vi "correctwaveformsizetemp.vi"(0 "new sampling frequency (Hz)":dbl, 1 "start":bool, 2 "reference waveforms to":string, 3 "Analog waveforms in":waveform(dbl)[](array[waveform]), 4 "stop":bool, 5 "Digital waveforms in":digitalwaveform[](array[waveform])) -> (6 "analog wf out":waveform(dbl)[](array[waveform]), 7 "Digital wf out":digitalwaveform[](array[waveform]), 8 "measpoints":i32)   [LabVIEW 2015]
uses:
  generateRampedSquareWave.vi
  waveformformfile.vi
  <vilib>/Waveform/DWDTOps.llb/DWDT Digital Size.vi
  digitalwffromfile.vi
  <vilib>/Waveform/DWDTOps.llb/DWDT Analog to Digital.vi
  <vilib>/Waveform/DWDTOps.llb/DWDT Append Digital Samples.vi
  <vilib>/Waveform/DWDTOps.llb/DWDT Get Waveform Subset.vi
  <vilib>/Waveform/WDTOps.llb/WDT Get Waveform Subset DBL.vi
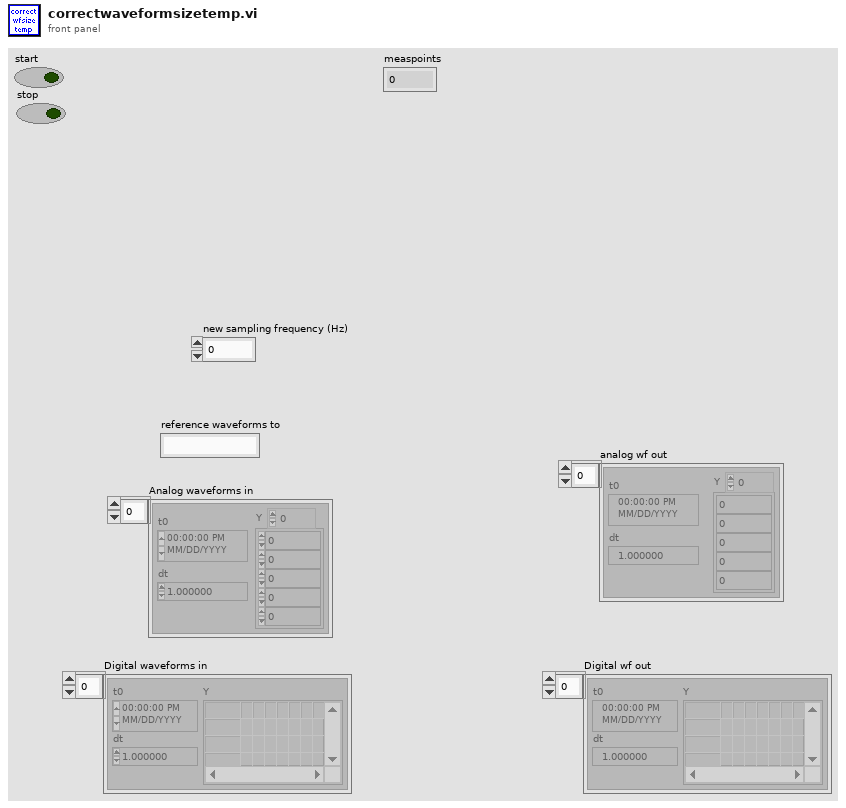
[diagram p1: front panel]
types:
  T1 = typedef "LVRectTypeDef.ctl" = cluster{"Left":i16, "Top":i16, "Right":i16, "Bottom":i16}
  T2 = cluster{"Xpixels":i32, "Vxminref":dbl, "Vxmaxref":dbl, "P":dbl, "Ypixels":i32, "Vyminref":dbl, "Vymaxref":dbl, "srate":sgl, "sAOxy":i32, "timeout":dbl, "type":string, "date":string, "time":string, "Colormap":u16, "Drawing Mode":u16, "Scanning Mode":u16, "square pixels":bool, "square matrix":bool, "Xpixels Img":i32, "Vx-min Img":dbl, "VX-max Img":dbl, "Ypixels Img":i32, "Vy-min Img":dbl, "Vy-max Img ":dbl, "Angle Img":dbl, "autoshutter":bool, "finite":bool, "cont":bool, "wavdet":bool, "measpoints":i32, "avpp":i32, "bufferAO":i32, "bufferAI":i32, "starttick":u32, "waveform":path, "Vx-ref":dbl, "Vy-ref":dbl, "refreshrate":dbl, "refreshbuffer":i32, "tt_cycles":i32, "motorref":refnum<k7>, "mirrorswitch":refnum<k7>, "sample mode":i32, "maxbufferAI":i32, "srateAODO":sgl, "bin":sgl, "Pel":sgl, "Angle draw":dbl, "srate Img":sgl, "ROIimg_plotbounds":T1, "auto OD":bool, "ODfilt":u16, "aAI":i32[], "aCI":i32[], "aAO":u32[], "aDO":u32[], "refwfsize":dbl, "Lifetime":bool, "Vz-Img":dbl, "Vz-ref":dbl, "Vz-reset":dbl, "AIoverride":bool, "aAS":u32[], "XYZstart":dbl[]}
  T3 = typedef "XYZStage.lvlib/XYZStage Configuration.ctl" = cluster{"VISA resource name":refnum<visa-resource-name>, "Timeout (3sec)":u32}
  T4 = cluster{"StageS":i32, "StageL":i32, "currmeas data dir":path, "image OD":u16, "contour OD":u16, "point OD":u16, "AOlines":tag[], "AIlines":tag[], "CI lines":tag[], "DO lines":tag[], "AO names":string[], "CI names":string[], "AI names":string[], "DO names":string[], "CIextensions":string[], "AIextensions":string[], "Voltage to Ygalvo":i32, "Voltage to Xgalvo":i32, "Voltage to patch":i32, "640 shutter":i32, "2P shutter":i32, "LT timestamp":u32, "Vp":i32, "Ip":i32, "camera trigger":i32, "master data dir":path, "voltage to Zpos":i32, "Vto2P":i32, "640 AO":i32, "488 AO":i32, "532 AO":i32, "640TTL":u32, "488TTL":u32, "532TTL":u32, "Device 1 sampleclock out":tag, "Device 1 Starttrigger out":tag, "Device 2 sampleclock in":tag, "Device 2 StartTrigger in ":tag, "2PODTTL":u32, "488 shutter":u32, "LCVR red":u32, "LCVR blue":u32, "Sutter Stage Config":T3}
  T5 = cluster{"AO parameters":cluster{"AOtab":dbl, "Repeats":dbl, "Cycles":dbl, "Start amplitude (V)":dbl, "Baseline (V)":dbl, "Step size (V)":dbl, "DC (%)":dbl, "Sampling frequency (Hz)":dbl, "Period (ms)":dbl, "Offset (V)":dbl, "Amplitude (V)":dbl, "Frequency":dbl, "Tri Repeats":dbl, "phase shift (ms)":dbl, "Pulses":dbl, "Matlab wave file":path, "Tri phase":dbl, "padding value":dbl}[], "DO parameters":cluster{"Digital DC (%)":dbl, "Digital phase":dbl, "Digital Freq (Hz)":dbl, "Sampling frequency (Hz)":dbl, "Digital time offset (s) ":dbl, "padding value":dbl, "matlab wave file":path, "DOtab":dbl}[]}
  T6 = cluster{"AOtab":dbl, "Repeats":dbl, "Cycles":dbl, "Start amplitude (V)":dbl, "Baseline (V)":dbl, "Step size (V)":dbl, "DC (%)":dbl, "Sampling frequency (Hz)":dbl, "Period (ms)":dbl, "Offset (V)":dbl, "Amplitude (V)":dbl, "Frequency":dbl, "Tri Repeats":dbl, "phase shift (ms)":dbl, "Pulses":dbl, "Matlab wave file":path, "Tri phase":dbl, "padding value":dbl}[]
  T7 = cluster{"AOtab":dbl, "Repeats":dbl, "Cycles":dbl, "Start amplitude (V)":dbl, "Baseline (V)":dbl, "Step size (V)":dbl, "DC (%)":dbl, "Sampling frequency (Hz)":dbl, "Period (ms)":dbl, "Offset (V)":dbl, "Amplitude (V)":dbl, "Frequency":dbl, "Tri Repeats":dbl, "phase shift (ms)":dbl, "Pulses":dbl, "Matlab wave file":path, "Tri phase":dbl, "padding value":dbl}
  T8 = cluster{"Digital DC (%)":dbl, "Digital phase":dbl, "Digital Freq (Hz)":dbl, "Sampling frequency (Hz)":dbl, "Digital time offset (s) ":dbl, "padding value":dbl, "matlab wave file":path, "DOtab":dbl}[]
  T9 = cluster{"Digital DC (%)":dbl, "Digital phase":dbl, "Digital Freq (Hz)":dbl, "Sampling frequency (Hz)":dbl, "Digital time offset (s) ":dbl, "padding value":dbl, "matlab wave file":path, "DOtab":dbl}
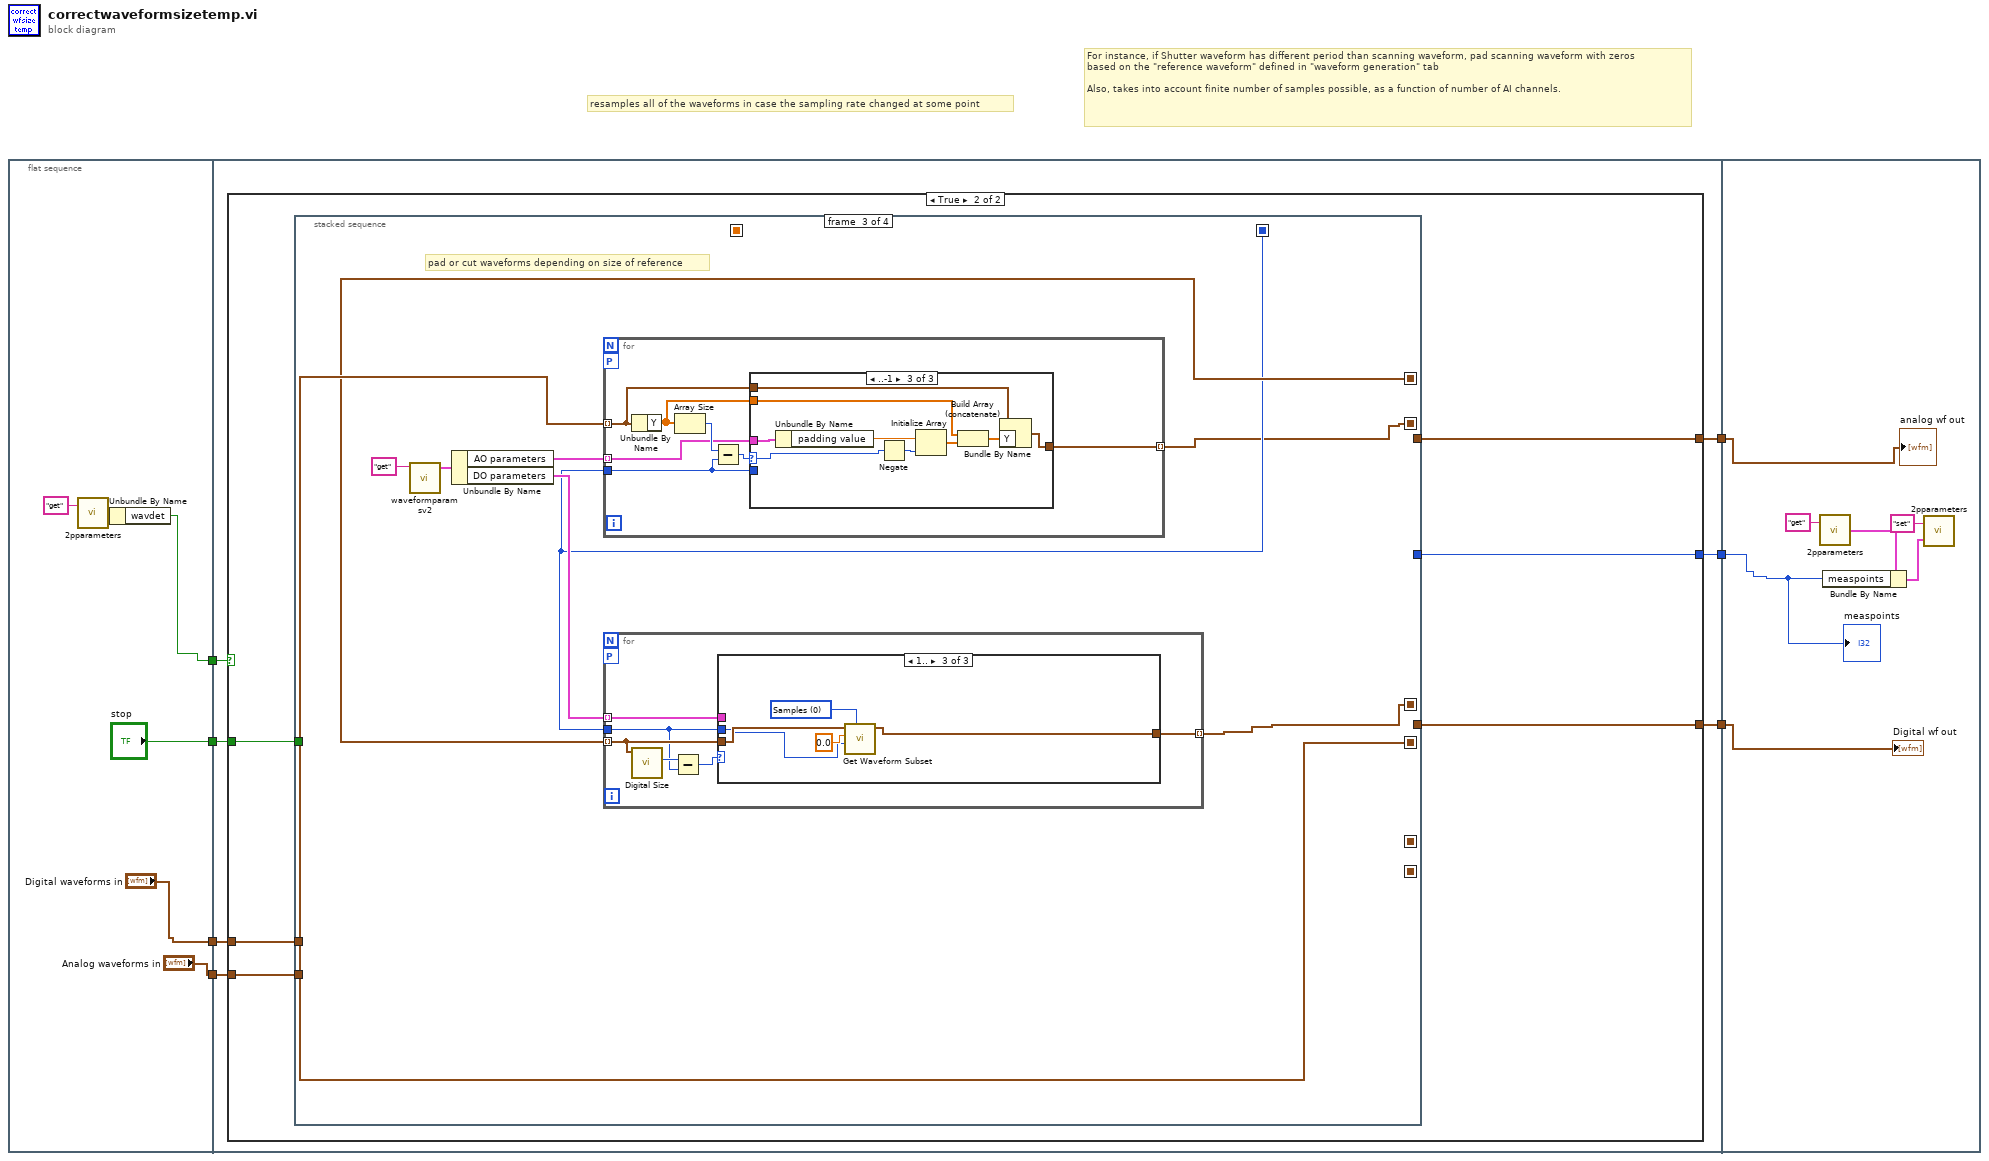
[diagram p0: block diagram]
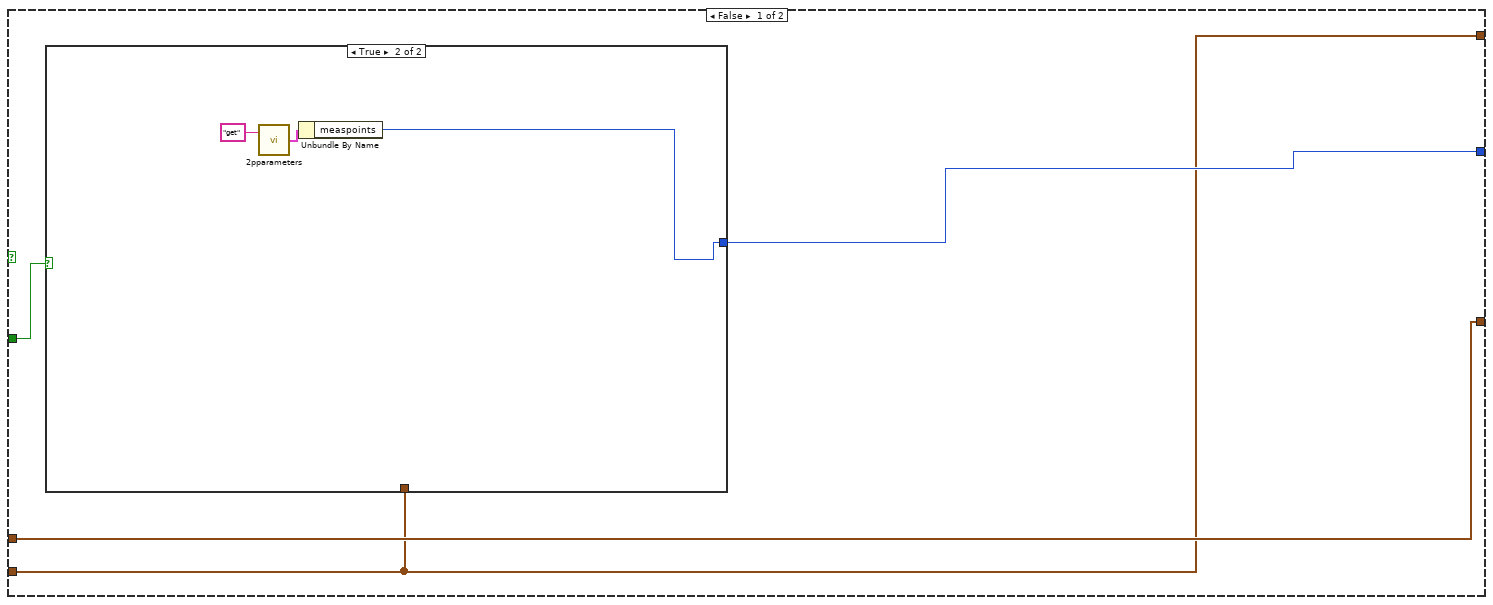
[diagram p2: hidden frame]
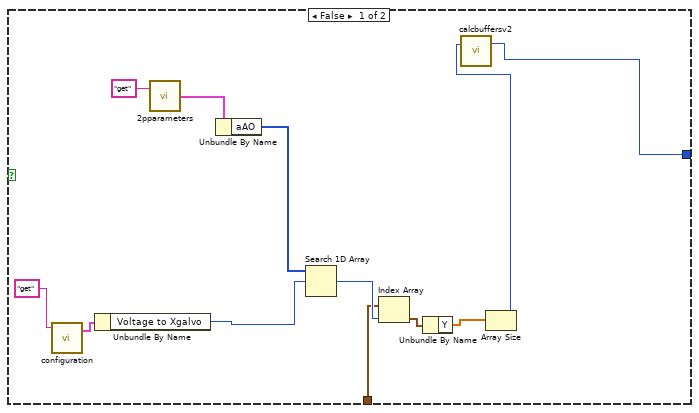
[diagram p3: hidden frame]
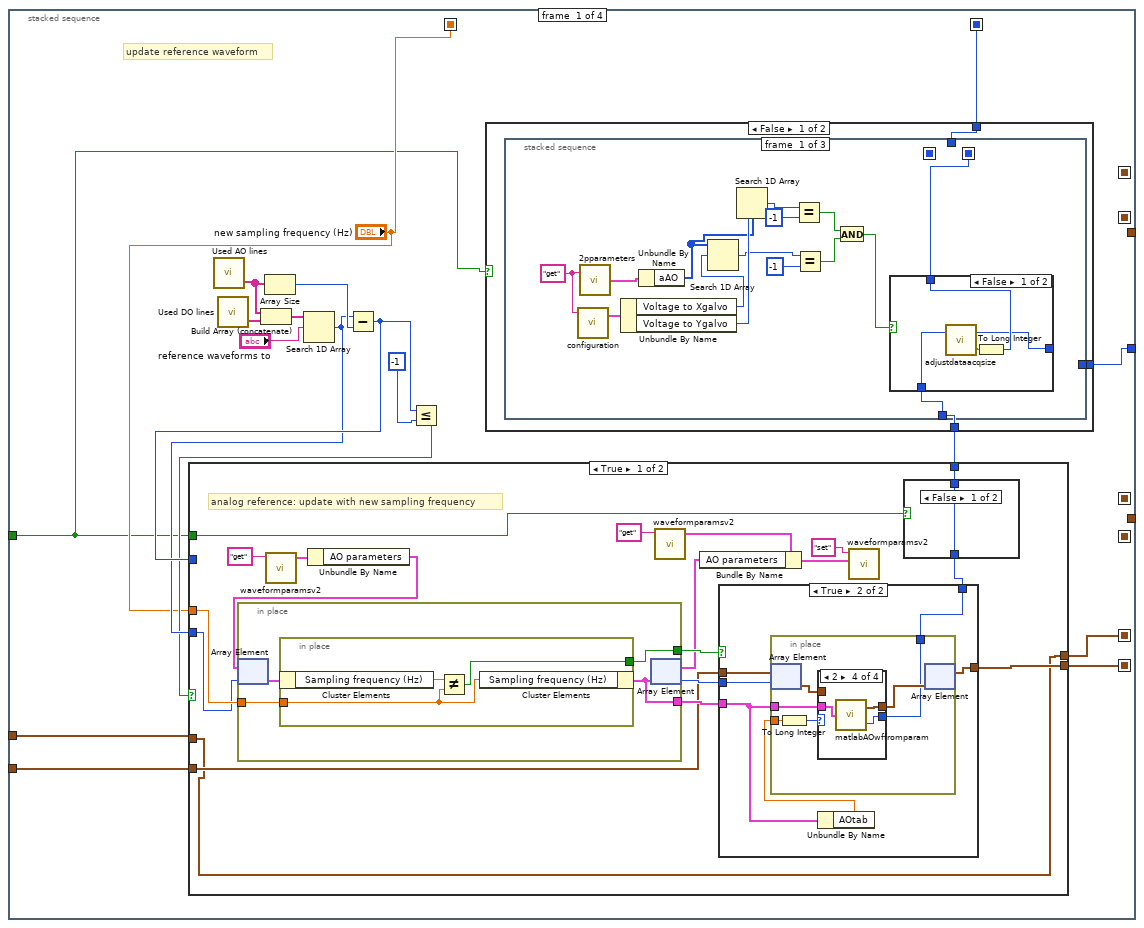
[diagram p4: hidden frame]
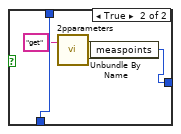
[diagram p5: hidden frame]
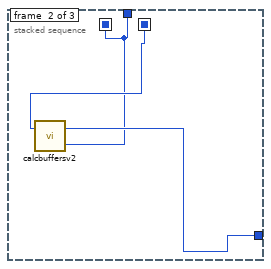
[diagram p6: hidden frame]
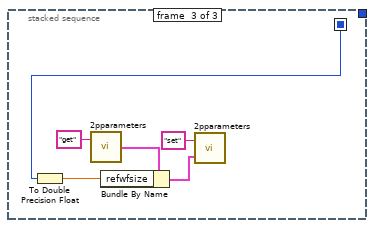
[diagram p7: hidden frame]
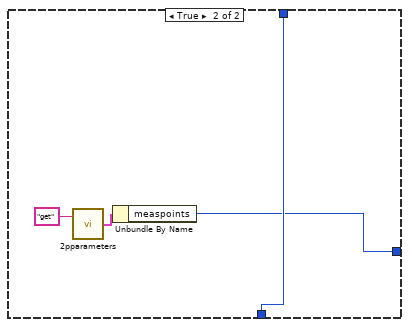
[diagram p8: hidden frame]
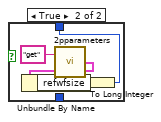
[diagram p9: hidden frame]
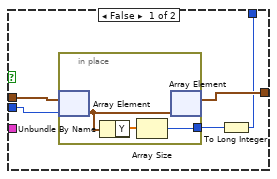
[diagram p10: hidden frame]
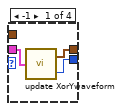
[diagram p11: hidden frame]
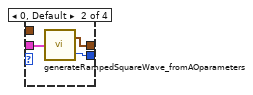
[diagram p12: hidden frame]
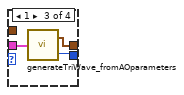
[diagram p13: hidden frame]
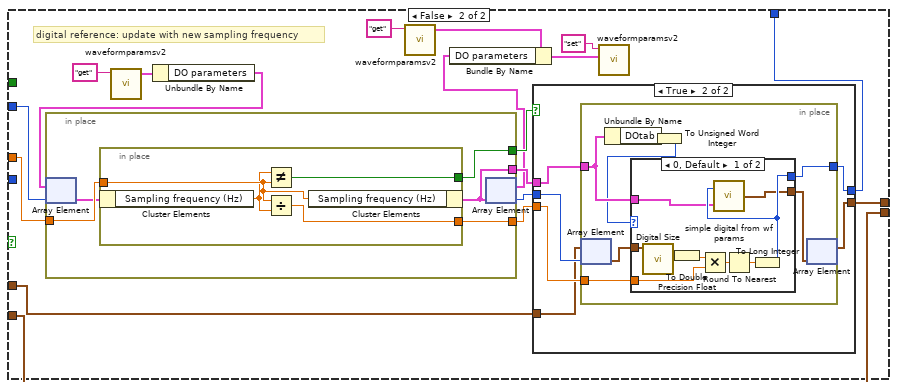
[diagram p14: hidden frame]
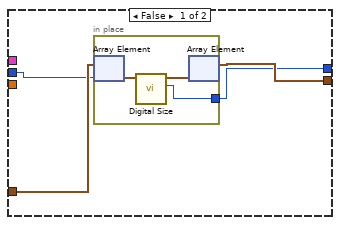
[diagram p15: hidden frame]
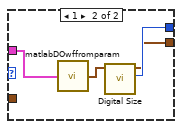
[diagram p16: hidden frame]
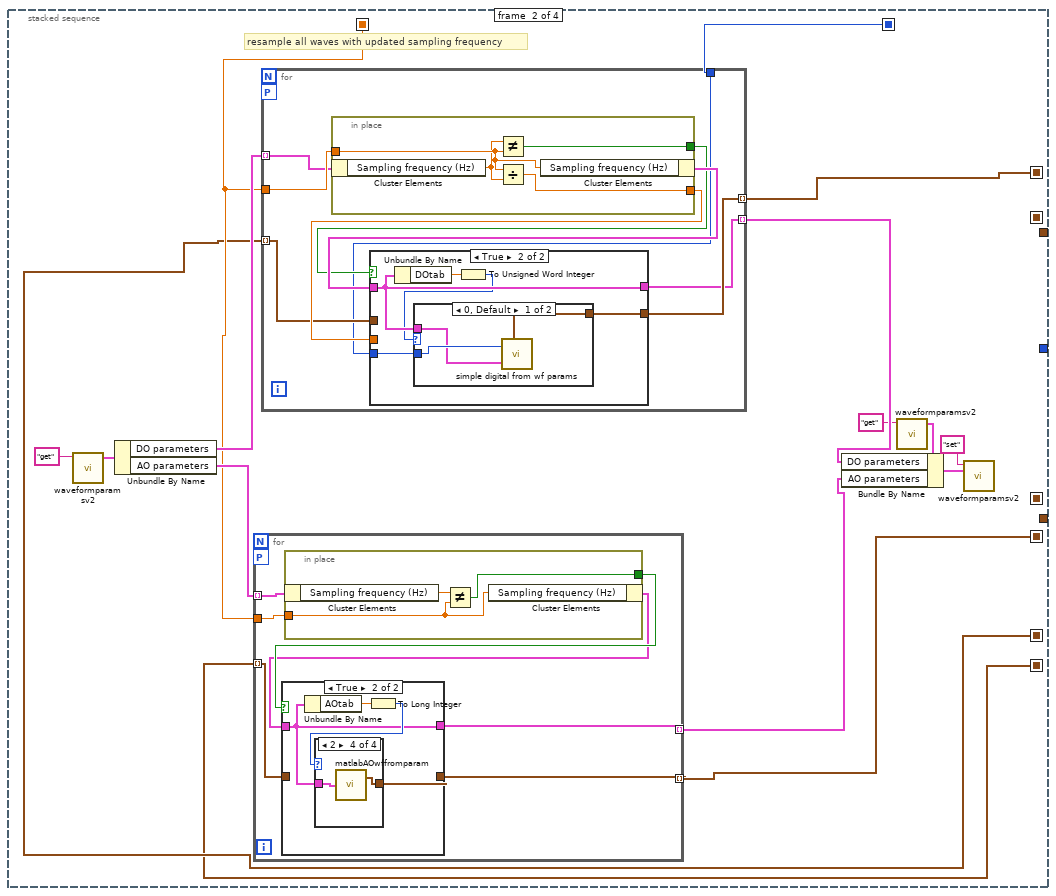
[diagram p17: hidden frame]
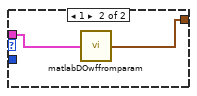
[diagram p19: hidden frame]
diagram:
  # "For instance, if Shutter waveform has different period than scanning waveform, pad scanning waveform with zeros\nbased on the \"reference waveform\" defined in \"waveform generation\" tab\n\nAlso, takes into account finite number of samples possible, as a function of number of AI channels."
  # "resamples all of the waveforms in case the sampling rate changed at some point"
  n1 = flat-sequence {
    tunnel: ["Digital waveforms in"] -> w7
    tunnel: ["Analog waveforms in"] -> w6
    tunnel: [w11] -> w5
    tunnel: ["stop"] -> w1
    tunnel: w7 -> [w19]
    tunnel: w6 -> [w18]
    tunnel: w5 -> [w15]
    tunnel: [w20] -> w4
    tunnel: [w17] -> w3
    tunnel: [w16] -> w2
    tunnel: w1 -> [w14]
    tunnel: w4 -> [w391]
    tunnel: w3 -> [w392]
    tunnel: w2 -> [w390]
    frame #0 {
      n2 = call "2pparameters.vi"("command"="get") -> ("params out"=w13:T2)  [unwired: 1 in]
      n3 = Unbundle By Name(w13) -> ("wavdet"=w11:bool)
    }
    frame #1 {
      n4 = case shown="True" w15 {
        tunnel: [w23 w45] -> w20
        tunnel: w19 -> [w24 w44]
        tunnel: w18 -> [w22 w43]
        tunnel: [w22 w42] -> w17
        tunnel: [w24 w41] -> w16
        tunnel: w14 -> [w21 w40]
        frame False {
          n5 = case shown="True" w21 {
            tunnel: [w31 w37] -> w23
            tunnel: w22 -> [w28 _]
            frame False {
              n6 = call "configuration.vi"("command"="get") -> ("config out"=w36:T4)  [unwired: 2 in, 1 out]
              n7 = Unbundle By Name(w36) -> ("Voltage to Xgalvo"=w32:i32)
              n8 = call "2pparameters.vi"("command"="get") -> ("params out"=w26:T2)  [unwired: 1 in]
              n9 = Unbundle By Name(w26) -> ("aAO"=w25:u32[])
              n10 = Search 1D Array(1D array=w25, element=w32) -> (index of element=w33:i32)  [unwired: 1 in]
              n11 = Index Array(array=w28, index=w33) -> (element=w29:waveform(dbl))
              n12 = Unbundle By Name(w29) -> ("Y"=w30:dbl[])
              n13 = Array Size(array=w30) -> (size(s)=w34:i32)
              n14 = call "calcbuffersv2.vi"("refsize"=w34) -> ("# of frames"=w31:i32)  [unwired: 1 in, 1 out]
            }
            frame True {
              n15 = call "2pparameters.vi"("command"="get") -> ("params out"=w38:T2)  [unwired: 1 in]
              n16 = Unbundle By Name(w38) -> ("measpoints"=w37:i32)
            }
          }
        }
        frame True {
          n17 = stacked-sequence {
            seq-local: [w47 _ _ _] -> [_ w233 w293 w353]
            seq-local: ["new sampling frequency (Hz)" _ _ _] -> [_ w230 _ _]
            seq-local: [w53 _ _ _] -> [_ w228 _ _]
            seq-local: [w52 _ _ _] -> [_ w229 _ _]
            seq-local: [_ w227 _ _] -> [_ _ w295 _]
            seq-local: [_ w226 _ _] -> [_ _ w294 _]
            seq-local: [_ _ w292 _] -> [_ _ _ w350]
            seq-local: [_ _ w291 _] -> [_ _ _ w349]
            tunnel: [w48 _ _ _] -> w45
            tunnel: w44 -> [w50 _ _ _]
            tunnel: w43 -> [w49 _ _ _]
            tunnel: [_ _ _ w352] -> w42
            tunnel: [_ _ _ w351] -> w41
            tunnel: w40 -> [w46 _ _ _]
            frame #0 {
              # "update reference waveform"
              n18 = call "Used AO lines.vi"() -> ("used AO names"=w58:string[])  [unwired: 2 in, 1 out]
              n19 = call "Used DO lines.vi"() -> ("used DO names"=w56:string[])  [unwired: 2 in, 1 out]
              n20 = Build Array (concatenate)(w58, w56) -> (w57:string[])
              n21 = Array Size(array=w58) -> (size(s)=w63:i32)
              n22 = Search 1D Array(1D array=w57, element="reference waveforms to") -> (index of element=w60:i32)  [unwired: 1 in]
              n23 = Subtract(x=w60, y=w63) -> (x-y=w61:i32)
              n24 = Less Or Equal?(x=w61, y=-1) -> (x <= y?=w59:bool)
              n25 = case shown="True" w59 {
                tunnel: w60 -> [w117 _]
                tunnel: w61 -> [_ w169]
                tunnel: "new sampling frequency (Hz)" -> [w118 w176]
                tunnel: [w105 w170] -> w51
                tunnel: w49 -> [w108 w168]
                tunnel: [w107 w168] -> w53
                tunnel: w50 -> [w106 w167]
                tunnel: [w106 w166] -> w52
                tunnel: w46 -> [w103 _]
                frame True {
                  # "analog reference: update with new sampling frequency"
                  n26 = call "waveformparamsv2.vi"("command"="get") -> ("Params out"=w121:T5)  [unwired: 4 in, 2 out]
                  n27 = Unbundle By Name(w121) -> ("AO parameters"=w119:T6)
                  n28 = in-place {
                    in-place-border: w118 -> [w129]
                    in-place-border: [w128] -> w116
                    in-place-border: [w127] -> w115
                    n29 = in-place-array #1(w119, w117) -> (w130:T7)
                    n30 = in-place {
                      in-place-border: w129 -> [w132]
                      in-place-border: [w131] -> w128
                      n31 = in-place-cluster #2(w130) -> ("Sampling frequency (Hz)"=w133:dbl)
                      n32 = Not Equal?(x=w133, y=w132) -> (x != y?=w131:bool)
                      n33 = in-place-cluster #2("Sampling frequency (Hz)"=w132) -> (w127:T7)
                    }
                    n34 = in-place-array #1(w127) -> (w110:T6, w114:i32)
                  }
                  n35 = call "waveformparamsv2.vi"("command"="get") -> ("Params out"=w111:T5)  [unwired: 4 in, 2 out]
                  n36 = Bundle By Name(cluster=w111, "AO parameters"=w110) -> (w109:T5)
                  n37 = case shown="True" w116 {
                    tunnel: w114 -> [w138 w147]
                    tunnel: w115 -> [_ w146]
                    tunnel: [w134 w142] -> w104
                    tunnel: w108 -> [w137 w144]
                    tunnel: [w136 w143] -> w107
                    frame False {
                      n38 = in-place {
                        in-place-border: [w140] -> w135
                        n39 = in-place-array #3(w137, w138) -> (w139:waveform(dbl))
                        n40 = Unbundle By Name(w139) -> ("Y"=w141:dbl[])
                        n41 = Array Size(array=w141) -> (size(s)=w140:i32)
                        n42 = in-place-array #3(w139) -> (w136:waveform(dbl)[])  [unwired: 1 out]
                      }
                      n43 = To Long Integer(number=w135) -> (32bit integer=w134:i32)
                    }
                    frame True {
                      n44 = Unbundle By Name(w146) -> ("AOtab"=w145:dbl)
                      n45 = in-place {
                        in-place-border: w146 -> [w152]
                        in-place-border: w145 -> [w150]
                        in-place-border: [w148] -> w142
                        n46 = in-place-array #4(w144, w147) -> (w149:waveform(dbl))
                        n47 = To Long Integer(number=w150) -> (32bit integer=w153:i32)
                        n48 = case shown="2" w153 {
                          tunnel: w152 -> [w156 w159 w162 w165]
                          tunnel: [w155 w158 w161 w164] -> w151
                          tunnel: w149 -> [_ _ _ _]
                          tunnel: [w154 w157 w160 w163] -> w148
                          frame -1 {
                            n49 = call "update XorYwaveform.vi"("AOparams"=w156) -> ("outputwave"=w155:waveform(dbl), "size"=w154:i32)
                          }
                          frame 0, Default {
                            n50 = call "generateRampedSquareWave_fromAOparameters.vi"("AO params"=w159) -> ("Waveform"=w158:waveform(dbl), "wflength"=w157:i32)
                          }
                          frame 1 {
                            n51 = call "generateTriWave_fromAOparameters.vi"("AO params"=w162) -> ("Waveform"=w161:waveform(dbl), "wfsize"=w160:i32)
                          }
                          frame 2 {
                            n52 = call "matlabAOwffromparam.vi"("Cluster"=w165) -> ("Waveform"=w164:waveform(dbl), "wfsize"=w163:i32)
                          }
                        }
                        n53 = in-place-array #4(w151) -> (w143:waveform(dbl)[])  [unwired: 1 out]
                      }
                    }
                  }
                  n54 = call "waveformparamsv2.vi"("command"="set", "Params in"=w109) -> ()  [unwired: 3 in, 3 out]
                  n55 = case shown="False" w103 {
                    tunnel: [w122 w123] -> w105
                    tunnel: w104 -> [w122 _]
                    frame False {
                    }
                    frame True {
                      n56 = call "2pparameters.vi"("command"="get") -> ("params out"=w125:T2)  [unwired: 1 in]
                      n57 = Unbundle By Name(w125) -> ("refwfsize"=w124:dbl)
                      n58 = To Long Integer(number=w124) -> (32bit integer=w123:i32)
                    }
                  }
                }
                frame False {
                  # "digital reference: update with new sampling frequency"
                  n59 = call "waveformparamsv2.vi"("command"="get") -> ("Params out"=w183:T5)  [unwired: 4 in, 2 out]
                  n60 = Unbundle By Name(w183) -> ("DO parameters"=w180:T8)
                  n61 = in-place {
                    in-place-border: [w188] -> w179
                    in-place-border: [w187] -> w178
                    in-place-border: [w186] -> w177
                    in-place-border: w176 -> [w185]
                    n62 = in-place-array #5(w180, w169) -> (w184:T9)
                    n63 = in-place {
                      in-place-border: w185 -> [w191]
                      in-place-border: [w192] -> w187
                      in-place-border: [w189] -> w186
                      n64 = in-place-cluster #6(w184) -> ("Sampling frequency (Hz)"=w190:dbl)
                      n65 = Not Equal?(x=w190, y=w191) -> (x != y?=w192:bool)
                      n66 = Divide(x=w191, y=w190) -> (x/y=w189:dbl)
                      n67 = in-place-cluster #6("Sampling frequency (Hz)"=w191) -> (w188:T9)
                    }
                    n68 = in-place-array #5(w188) -> (w171:T8, w181:i32)
                  }
                  n69 = call "waveformparamsv2.vi"("command"="get") -> ("Params out"=w173:T5)  [unwired: 4 in, 2 out]
                  n70 = Bundle By Name(cluster=w173, "DO parameters"=w171) -> (w172:T5)
                  n71 = case shown="True" w178 {
                    tunnel: w181 -> [w195 w202]
                    tunnel: w179 -> [_ w205]
                    tunnel: w177 -> [_ w204]
                    tunnel: [w193 w203] -> w170
                    tunnel: w167 -> [w196 w201]
                    tunnel: [w194 w200] -> w166
                    frame False {
                      n72 = in-place {
                        in-place-border: [w197] -> w193
                        n73 = in-place-array #7(w196, w195) -> (w199:digitalwaveform)
                        n74 = call-poly <vilib>:"Digital Size.vi"("digital waveform in"=w199) -> ("number of samples"=w197:i32, "digital waveform out"=w198:digitalwaveform)  [unwired: 7 in, 2 out]
                        n75 = in-place-array #7(w198) -> (w194:digitalwaveform[])  [unwired: 1 out]
                      }
                    }
                    frame True {
                      n76 = in-place {
                        in-place-border: w205 -> [w210]
                        in-place-border: w204 -> [w212]
                        in-place-border: [w211] -> w203
                        n77 = in-place-array #8(w201, w202) -> (w208:digitalwaveform)
                        n78 = Unbundle By Name(w210) -> ("DOtab"=w209:dbl)
                        n79 = To Unsigned Word Integer(number=w209) -> (unsigned 16bit integer=w206:u16)
                        n80 = case shown="0, Default" w206 {
                          tunnel: w212 -> [w219 _]
                          tunnel: [w216 w223] -> w211
                          tunnel: [w215 w222] -> w207
                          tunnel: w210 -> [w214 w225]
                          tunnel: w208 -> [w213 _]
                          frame 0, Default {
                            n81 = call-poly <vilib>:"Digital Size.vi"("digital waveform in"=w213) -> ("number of samples"=w221:i32)  [unwired: 7 in, 3 out]
                            n82 = To Double Precision Float(number=w221) -> (double precision float=w220:dbl)
                            n83 = Multiply(x=w220, y=w219) -> (x*y=w218:dbl)
                            n84 = Round To Nearest(number=w218) -> (nearest integer value=w217:dbl)
                            n85 = To Long Integer(number=w217) -> (32bit integer=w216:i32)
                            n86 = call "simple digital from wf params.vi"("waveform params"=w214, "number of samples"=w216) -> ("digital waveform"=w215:digitalwaveform)
                          }
                          frame 1 {
                            n87 = call "matlabDOwffromparam.vi"("waveform params"=w225) -> ("digital waveform"=w224:digitalwaveform)
                            n88 = call-poly <vilib>:"Digital Size.vi"("digital waveform in"=w224) -> ("number of samples"=w223:i32, "digital waveform out"=w222:digitalwaveform)  [unwired: 7 in, 2 out]
                          }
                        }
                        n89 = in-place-array #8(w207) -> (w200:digitalwaveform[])  [unwired: 1 out]
                      }
                    }
                  }
                  n90 = call "waveformparamsv2.vi"("command"="set", "Params in"=w172) -> ()  [unwired: 3 in, 3 out]
                }
              }
              n91 = case shown="False" w46 {
                tunnel: w51 -> [w66 w102]
                tunnel: [w65 w99] -> w48
                tunnel: [w64 w102] -> w47
                frame False {
                  n92 = stacked-sequence {
                    seq-local: [w67 _ _] -> [_ w92 _]
                    seq-local: [_ w90 _] -> [_ _ w93]
                    tunnel: w66 -> [w81 _ _]
                    tunnel: [_ w90 _] -> w64
                    tunnel: [_ w91 _] -> w65
                    frame #0 {
                      w79 = "get" ("command")
                      n93 = call "configuration.vi"("command"=w79) -> ("config out"=w78:T4)  [unwired: 2 in, 1 out]
                      n94 = call "2pparameters.vi"("command"=w79) -> ("params out"=w80:T2)  [unwired: 1 in]
                      n95 = Unbundle By Name(w78) -> ("Voltage to Xgalvo"=w77:i32, "Voltage to Ygalvo"=w76:i32)
                      n96 = Unbundle By Name(w80) -> ("aAO"=w75:u32[])
                      n97 = Search 1D Array(1D array=w75, element=w77) -> (index of element=w71:i32)  [unwired: 1 in]
                      n98 = Search 1D Array(1D array=w75, element=w76) -> (index of element=w74:i32)  [unwired: 1 in]
                      n99 = Equal?(x=w74, y=-1) -> (x = y?=w70:bool)
                      n100 = Equal?(x=w71, y=-1) -> (x = y?=w69:bool)
                      n101 = And(x=w70, y=w69) -> (x .and. y?=w68:bool)
                      n102 = case shown="False" w68 {
                        tunnel: w81 -> [w85 w89]
                        tunnel: [w83 w89] -> w67
                        tunnel: [w82 w86] -> _
                        frame False {
                          n103 = call "adjustdataacqsize.vi"("waveform size in"=w85) -> ("waveform size out"=w84:dbl, "# of points"=w82:i32)  [unwired: 1 in]
                          n104 = To Long Integer(number=w84) -> (32bit integer=w83:i32)
                        }
                        frame True {
                          n105 = call "2pparameters.vi"("command"="get") -> ("params out"=w87:T2)  [unwired: 1 in]
                          n106 = Unbundle By Name(w87) -> ("measpoints"=w86:i32)
                        }
                      }
                    }
                    frame #1 {
                      n107 = call "calcbuffersv2.vi"("refsize"=w92) -> ("wfsize"=w90:i32, "# of frames"=w91:i32)  [unwired: 1 in]
                    }
                    frame #2 {
                      n108 = To Double Precision Float(number=w93) -> (double precision float=w98:dbl)
                      n109 = call "2pparameters.vi"("command"="get") -> ("params out"=w96:T2)  [unwired: 1 in]
                      n110 = Bundle By Name(cluster=w96, "refwfsize"=w98) -> (w97:T2)
                      n111 = call "2pparameters.vi"("Params in"=w97, "command"="set") -> ()  [unwired: 1 out]
                    }
                  }
                }
                frame True {
                  n112 = call "2pparameters.vi"("command"="get") -> ("params out"=w100:T2)  [unwired: 1 in]
                  n113 = Unbundle By Name(w100) -> ("measpoints"=w99:i32)
                }
              }
            }
            frame #1 {
              # "resample all waves with updated sampling frequency"
              n114 = call "waveformparamsv2.vi"("command"="get") -> ("Params out"=w241:T5)  [unwired: 4 in, 2 out]
              n115 = Unbundle By Name(w241) -> ("DO parameters"=w232:T8, "AO parameters"=w231:T6)
              n116 = for {
                tunnel: w231 -> [w273] mode=indexing
                workers-P: _ -> [_]
                tunnel: w230 -> [w272]
                tunnel: [w269] -> w227 mode=indexing
                tunnel: [w268] -> w234 mode=indexing
                tunnel: w228 -> [w267] mode=indexing
                n117 = in-place {
                  in-place-border: w272 -> [w289]
                  in-place-border: [w288] -> w271
                  n118 = in-place-cluster #9(w273) -> ("Sampling frequency (Hz)"=w290:dbl)
                  n119 = Not Equal?(x=w290, y=w289) -> (x != y?=w288:bool)
                  n120 = in-place-cluster #9("Sampling frequency (Hz)"=w289) -> (w270:T7)
                }
                n121 = case shown="True" w271 {
                  tunnel: w270 -> [w275 w277]
                  tunnel: [w275 w277] -> w268
                  tunnel: [w274 w276] -> w269
                  tunnel: w267 -> [w274 _]
                  frame False {
                  }
                  frame True {
                    n122 = Unbundle By Name(w277) -> ("AOtab"=w279:dbl)
                    n123 = To Long Integer(number=w279) -> (32bit integer=w278:i32)
                    n124 = case shown="2" w278 {
                      tunnel: w277 -> [w281 w283 w285 w286]
                      tunnel: [w280 w282 w284 w287] -> w276
                      frame -1 {
                        n125 = call "update XorYwaveform.vi"("AOparams"=w281) -> ("outputwave"=w280:waveform(dbl))  [unwired: 1 out]
                      }
                      frame 0, Default {
                        n126 = call "generateRampedSquareWave_fromAOparameters.vi"("AO params"=w283) -> ("Waveform"=w282:waveform(dbl))  [unwired: 1 out]
                      }
                      frame 1 {
                        n127 = call "generateTriWave_fromAOparameters.vi"("AO params"=w285) -> ("Waveform"=w284:waveform(dbl))  [unwired: 1 out]
                      }
                      frame 2 {
                        n128 = call "matlabAOwffromparam.vi"("Cluster"=w286) -> ("Waveform"=w287:waveform(dbl))  [unwired: 1 out]
                      }
                    }
                  }
                }
              }
              n129 = for {
                tunnel: w230 -> [w250]
                tunnel: w232 -> [w249] mode=indexing
                tunnel: w229 -> [w244] mode=indexing
                tunnel: [w245] -> w226 mode=indexing
                tunnel: [w243] -> w239 mode=indexing
                workers-P: _ -> [_]
                tunnel: w233 -> [w242]
                n130 = in-place {
                  in-place-border: w250 -> [w265]
                  in-place-border: [w266] -> w247
                  in-place-border: [w263] -> w246
                  n131 = in-place-cluster #10(w249) -> ("Sampling frequency (Hz)"=w264:dbl)
                  n132 = Not Equal?(x=w264, y=w265) -> (x != y?=w266:bool)
                  n133 = Divide(x=w265, y=w264) -> (x/y=w263:dbl)
                  n134 = in-place-cluster #10("Sampling frequency (Hz)"=w265) -> (w248:T9)
                }
                n135 = case shown="True" w247 {
                  tunnel: w248 -> [w251 w254]
                  tunnel: w246 -> [_ _]
                  tunnel: [w252 w257] -> w245
                  tunnel: w244 -> [w252 _]
                  tunnel: [w251 w254] -> w243
                  tunnel: w242 -> [_ w256]
                  frame False {
                  }
                  frame True {
                    n136 = Unbundle By Name(w254) -> ("DOtab"=w255:dbl)
                    n137 = To Unsigned Word Integer(number=w255) -> (unsigned 16bit integer=w253:u16)
                    n138 = case shown="0, Default" w253 {
                      tunnel: [w260 w261] -> w257
                      tunnel: w256 -> [w259 _]
                      tunnel: w254 -> [w258 w262]
                      frame 0, Default {
                        n139 = call "simple digital from wf params.vi"("waveform params"=w258, "number of samples"=w259) -> ("digital waveform"=w260:digitalwaveform)
                      }
                      frame 1 {
                        n140 = call "matlabDOwffromparam.vi"("waveform params"=w262) -> ("digital waveform"=w261:digitalwaveform)
                      }
                    }
                  }
                }
              }
              n141 = call "waveformparamsv2.vi"("command"="get") -> ("Params out"=w236:T5)  [unwired: 4 in, 2 out]
              n142 = Bundle By Name(cluster=w236, "DO parameters"=w239, "AO parameters"=w234) -> (w235:T5)
              n143 = call "waveformparamsv2.vi"("command"="set", "Params in"=w235) -> ()  [unwired: 3 in, 3 out]
            }
            frame #2 {
              # "pad or cut waveforms depending on size of reference"
              n144 = call "waveformparamsv2.vi"("command"="get") -> ("Params out"=w297:T5)  [unwired: 4 in, 2 out]
              n145 = Unbundle By Name(w297) -> ("AO parameters"=w299:T6, "DO parameters"=w298:T8)
              n146 = for {
                tunnel: w295 -> [w330] mode=indexing
                tunnel: [w329] -> w292 mode=indexing
                workers-P: _ -> [_]
                tunnel: w293 -> [w331]
                tunnel: w299 -> [w328] mode=indexing
                n147 = Unbundle By Name(w330) -> ("Y"=w327:dbl[])
                n148 = Array Size(array=w327) -> (size(s)=w332:i32)
                n149 = Subtract(x=w332, y=w331) -> (x-y=w333:i32)
                n150 = case shown="..-1" w333 {
                  selector: w333 -> [_ _ w346]
                  tunnel: [w334 w338 w339] -> w329
                  tunnel: w331 -> [w336 _ _]
                  tunnel: w330 -> [w337 w338 w340]
                  tunnel: w328 -> [_ _ w347]
                  tunnel: w327 -> [_ _ w343]
                  frame 1.. {
                    w335 = u16 0 items=["Samples", "Relative Time"] ("start/duration format")
                    n151 = call-poly <vilib>:"Get Waveform Subset.vi"("start/duration format"=w335, "duration"=w336, "waveform in"=w337) -> ("waveform out"=w334:waveform(dbl))  [unwired: 3 in, 3 out]
                  }
                  frame 0 {
                  }
                  frame ..-1 {
                    n152 = Unbundle By Name(w347) -> ("padding value"=w344:dbl)
                    n153 = Negate(x=w346) -> (-x=w345:i32)
                    n154 = Initialize Array(w344, w345) -> (w342:dbl[])
                    n155 = Build Array (concatenate)(w343, w342) -> (w341:dbl[])
                    n156 = Bundle By Name(cluster=w340, "Y"=w341) -> (w339:waveform(dbl))
                  }
                }
              }
              n157 = for {
                tunnel: w294 -> [w302] mode=indexing
                tunnel: w298 -> [w304] mode=indexing
                tunnel: [w301] -> w291 mode=indexing
                tunnel: w293 -> [w300]
                workers-P: _ -> [_]
                n158 = call-poly <vilib>:"Digital Size.vi"("digital waveform in"=w302) -> ("number of samples"=w303:i32)  [unwired: 7 in, 3 out]
                n159 = Subtract(x=w303, y=w300) -> (x-y=w305:i32)
                n160 = case shown="1.." w305 {
                  selector: w305 -> [w318 _ _]
                  tunnel: w300 -> [_ _ w323]
                  tunnel: w304 -> [w320 _ _]
                  tunnel: w302 -> [w312 w321 w325]
                  tunnel: [w310 w321 w326] -> w301
                  frame ..-1 {
                    w306 = u16 0 items=["unsigned binary", "offset binary", "2's complement"] ("data format (offset binary)")
                    n161 = Unbundle By Name(w320) -> ("Sampling frequency (Hz)"=w315:dbl, "padding value"=w319:dbl)
                    n162 = Negate(x=w318) -> (-x=w317:i32)
                    n163 = Initialize Array(w319, w317) -> (w316:dbl[])
                    n164 = Reciprocal(x=w315) -> (1/x=w314:dbl)
                    n165 = Bundle By Name("Y"=w316, "dt"=w314) -> (w313:waveform(dbl))  [unwired: 1 in]
                    n166 = call-poly <vilib>:"Analog to Digital.vi"("data format (offset binary)"=w306, "compress digital (T)"=TRUE, "full-scale range (pk-pk)"=1.0, "resolution (16 bit)"=1, "analog waveform"=w313) -> ("digital waveform"=w311:digitalwaveform)  [unwired: 3 in, 3 out]
                    n167 = call-poly <vilib>:"Append Digital Samples.vi"("digital waveform B"=w311, "digital waveform A"=w312) -> ("digital waveform out"=w310:digitalwaveform)  [unwired: 8 in, 1 out]
                  }
                  frame 0 {
                  }
                  frame 1.. {
                    w322 = u16 0 items=["Samples", "Relative Time"] ("start/duration format")
                    n168 = call-poly <vilib>:"Get Waveform Subset.vi"("start/duration format"=w322, "duration"=w323, "start samples/time"=0.0, "waveform in"=w325) -> ("waveform out"=w326:digitalwaveform)  [unwired: 2 in, 3 out]
                  }
                }
              }
            }
            frame #3 {
              # "pad or cut waveforms depending on size of reference"
              n169 = case shown="True" "start" {
                tunnel: w353 -> [_ _]
                tunnel: [w355 w359] -> w352
                tunnel: [w354 w358] -> w351
                tunnel: w350 -> [w355 w357]
                tunnel: w349 -> [w354 w356]
                frame False {
                }
                frame True {
                  n170 = call "waveformparamsv2.vi"("command"="get") -> ("Params out"=w361:T5)  [unwired: 4 in, 2 out]
                  n171 = Unbundle By Name(w361) -> ("AO parameters"=w363:T6, "DO parameters"=w362:T8)
                  n172 = for {
                    tunnel: w357 -> [w389] mode=indexing
                    tunnel: [w388] -> w359 mode=indexing
                    workers-P: _ -> [_]
                    tunnel: w363 -> [w387] mode=indexing
                    n173 = Unbundle By Name(w389) -> ("Y"=w386:dbl[])
                    n174 = Unbundle By Name(w387) -> ("padding value"=w385:dbl)
                    n175 = call "2pparameters.vi"("command"="get") -> ("params out"=w381:T2)  [unwired: 1 in]
                    n176 = Unbundle By Name(w381) -> ("bufferAO"=w380:i32)
                    n177 = Initialize Array(w385, w380) -> (w384:dbl[])
                    n178 = Build Array (concatenate)(w386, w384) -> (w383:dbl[])
                    n179 = Bundle By Name(cluster=w389, "Y"=w383) -> (w388:waveform(dbl))
                  }
                  n180 = for {
                    tunnel: w356 -> [w378] mode=indexing
                    tunnel: w362 -> [w379] mode=indexing
                    tunnel: [w377] -> w358 mode=indexing
                    workers-P: _ -> [_]
                    w367 = u16 0 items=["unsigned binary", "offset binary", "2's complement"] ("data format (offset binary)")
                    n181 = call "2pparameters.vi"("command"="get") -> ("params out"=w366:T2)  [unwired: 1 in]
                    n182 = Unbundle By Name(w379) -> ("Sampling frequency (Hz)"=w374:dbl, "padding value"=w376:dbl)
                    n183 = Unbundle By Name(w366) -> ("bufferAO"=w364:i32)
                    n184 = Initialize Array(w376, w364) -> (w375:dbl[])
                    n185 = Reciprocal(x=w374) -> (1/x=w373:dbl)
                    n186 = Bundle By Name("Y"=w375, "dt"=w373) -> (w372:waveform(dbl))  [unwired: 1 in]
                    n187 = call-poly <vilib>:"Analog to Digital.vi"("data format (offset binary)"=w367, "compress digital (T)"=TRUE, "full-scale range (pk-pk)"=1.0, "resolution (16 bit)"=1, "analog waveform"=w372) -> ("digital waveform"=w371:digitalwaveform)  [unwired: 3 in, 3 out]
                    n188 = call-poly <vilib>:"Append Digital Samples.vi"("digital waveform B"=w371, "digital waveform A"=w378) -> ("digital waveform out"=w377:digitalwaveform)  [unwired: 8 in, 1 out]
                  }
                }
              }
            }
          }
        }
      }
    }
    frame #2 {
      n189 = call "2pparameters.vi"("command"="get") -> ("params out"=w395:T2)  [unwired: 1 in]
      n190 = Bundle By Name(cluster=w395, "measpoints"=w391) -> (w396:T2)
      n191 = call "2pparameters.vi"("Params in"=w396, "command"="set") -> ()  [unwired: 1 out]
      "analog wf out" <- w392
      "Digital wf out" <- w390
      "measpoints" <- w391
    }
  }
